vi "Send Command.vi"(8 "error in (no error)":errorcluster, 10 "Consumer Queues in":T1, 11 "Generic Command in":refnum<class "Generic Command.lvclass">) -> (0 "error out":errorcluster, 2 "Consumer Queues out":T1)   [LabVIEW 2019, in "Generic Command.lvclass"]
uses:
  Generic Command.lvclass
  TS Framework/Consumer Queues.ctl
  UI Process/Generic UI Command/Generic UI Process Command.lvclass
  DAC Process/Generic DAC Command/Generic DAC Process Command.lvclass
  Trig Process/Generic Trig Command/Generic Trig Process Command.lvclass
  TS Framework/TS Framework.lvlib
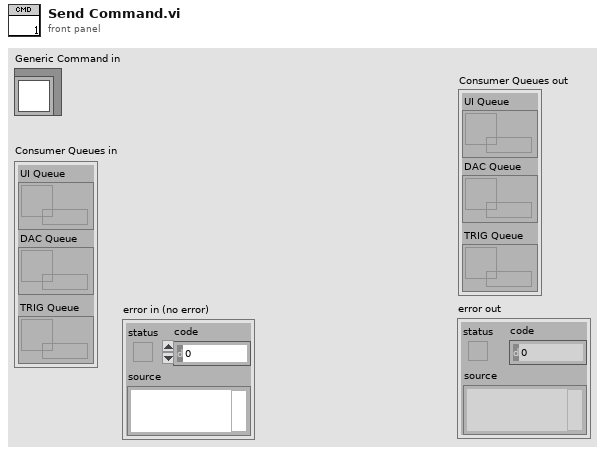
[diagram p1: front panel]
types:
  T1 = typedef "TS Framework.lvlib/Consumer Queues.ctl" = cluster{"UI Queue":refnum<queue>, "DAC Queue":refnum<queue>, "TRIG Queue":refnum<queue>}
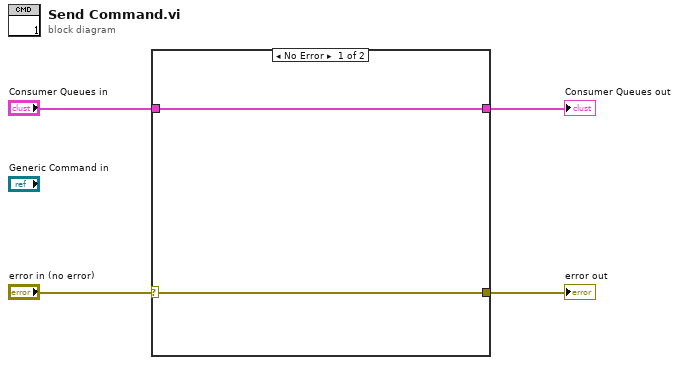
[diagram p0: block diagram]
diagram:
  n1 = case shown="No Error" "error in (no error)" {
    selector: "error in (no error)" -> [w6 w8]
    tunnel: [w6 w8] -> w3
    tunnel: "Consumer Queues in" -> [w5 w7]
    tunnel: [w5 w7] -> w1
    frame No Error {
    }
    frame Error {
    }
  }
  "error out" <- w3
  "Consumer Queues out" <- w1
